vi "S2C_FORNAX_Proc_SendExit.vi"(8 "Error In":errorcluster, 11 "Refs":string[][](array[string])) -> (0 "Error Out":errorcluster)   [LabVIEW 2015]
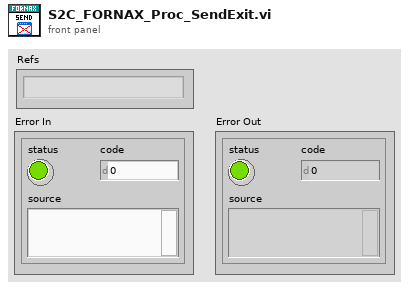
[diagram p1: front panel]
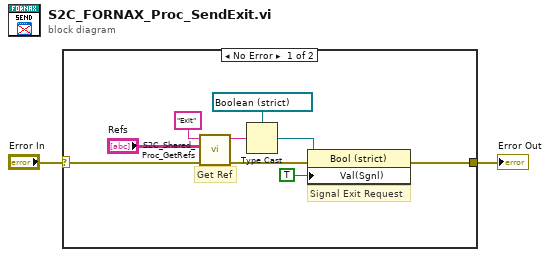
[diagram p0: block diagram]
diagram:
  n1 = case shown="No Error" "Error In" {
    selector: "Error In" -> [w5 w12]
    tunnel: [w4 w12] -> w1
    frame No Error {
      # "Signal Exit Request"
      # "Get Ref"
      n2 = call "S2C_Shared_Proc_GetRefs.vi"("Error In"=w5, "Refs"="Refs", "Label"="Exit") -> ("Error Out"=w8:errorcluster, "Reference"=w10:string)  [unwired: 7 in]
      n3 = Type Cast(type=refnum<vi> refnum ("Exit"), x=w10) -> (*(type *) &x=w7:refnum<vi>)
      n4 = property class="Bool (strict)"(reference=w7, error in=w8, "Val(Sgnl)"=TRUE ("Value (Signaling)")) -> (error out=w4:errorcluster)  [unwired: 1 out]
    }
    frame Error {
    }
  }
  "Error Out" <- w1
